vi "DevB.Send Message.vi"   [LabVIEW 2018]
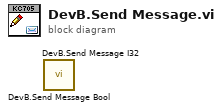
[diagram p0: block diagram]
diagram:
  n1 = call "DevB.Send Message Bool.vi"() -> ()  [unwired: 10 in, 2 out]
  n2 = call "DevB.Send Message I32.vi"() -> ()  [unwired: 10 in, 2 out]
